vi "subUpdateTypePaletteFile.vi"(8 "error in (no error)":errorcluster, 9 "Step Types Version":string, 11 "TypePalette .ini file location":path) -> (0 "error out":errorcluster)   [LabVIEW 2015, in "veristand-steps-codegen.lvlib"]
uses:
  veristand-steps-codegen.lvlib
  <vilib>/Utility/sysdir.llb/System Directory Type.ctl
  <vilib>/xml/Load XML File.vi
  <vilib>/xml/Close Reference(Node).vi
  <vilib>/xml/Close Reference(NNMap).vi
  <vilib>/xml/NI_XML.lvlib
  <resource>/objmgr/DOMUserDefRef.rc
  <vilib>/ni/Simple XML/Simple XML.lvlib
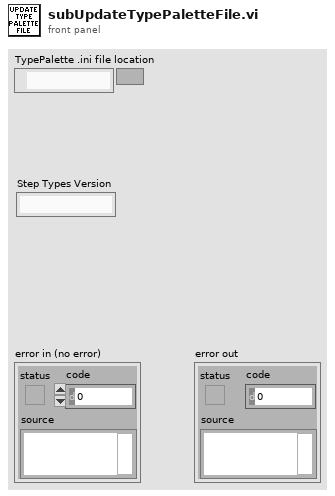
[diagram p1: front panel]
types:
  T1 = typedef "System Directory Type.ctl" = i32
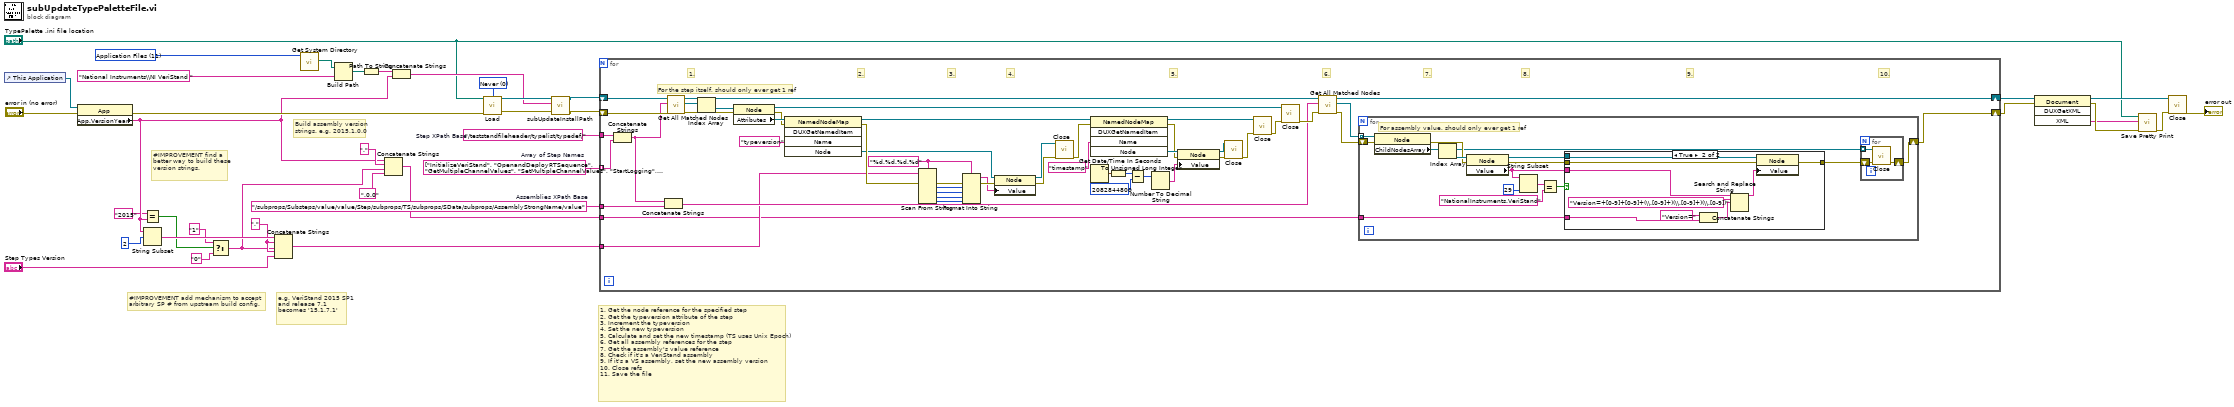
[diagram p0: block diagram]
diagram:
  w6 = "." ("string")
  w19 = T1 11 items=["User Home"=0, "User Desktop"=1, "User Documents"=2, "User Application Data"=3, "User Preferences"=4, "User Temporary"=5, "Public Documents"=6, "Public Application Data"=7, "Public Preferences"=8, "Public Cache"=13, "System Core Libraries"=9, "System Installed Libraries"=10, "Application Files"=11, "Boot Volume Root"=12] ("system directory type")
  w39 = "/subprops/Substeps/value/value/Step/subprops/TS/subprops/SData/subprops/AssemblyStrongName/value"  # Assemblies XPath Base
  w37 = string[] ["InitializeVeriStand", "OpenandDeployRTSequence", "GetMultipleChannelValues", "SetMultipleChannelValues", "StartLogging", "StopLogging", "StopVeriStand", "RunProject", "ConnectProject", "DisconnectProject", "UndeployProject", "RunStimulusProfileAsynch", "DeployProject", "OpenReferences", "GetAlarmState", "SetChannelValue", "GetAlarmList", "RunStimulusProfileBlocking", "SetAlarmState", "SetModelParameterValue", "CloseProject", "UpdateModelParametersFromFile", "GetChannelValue", "LimitTestChannelValue", "GetChannelFaultValue", "GetModelParameterValue", "ClearFault", "ClearAllFaults", "PauseRTSequence", "StopRTSequence", "GetSequenceState", "GetAllSequenceNames", "StartRTSequence", "AbortRTSequence", "GetSequenceReturnValue", "StartStimulusProfileSession", "RunRTSequenceAction", "CloseWorkspace", "OpenWorkspace", "SilentConnect", "SilentDisconnect", "OpenProject", "RunRTSequencePassFail", "RunRTSequenceNumericLimit", "SetChannelFaultValue", "StopVeristandGateway", "StartVeristand"]  # Array of Step Names
  w31 = "/teststandfileheader/typelist/typedef/"  # Step XPath Base
  w30 = 0 items=["Never", "Always", "Auto"] ("validate on load (Auto)")
  # "#IMPROVEMENT find a better way to build these version strings."
  # "Build assembly version\nstrings. e.g. 2015.1.0.0"
  # "#IMPROVEMENT add mechanism to accept\narbitrary SP # from upstream build config."
  # "e.g. VeriStand 2015 SP1 and release 7.1\nbecomes '15.1.7.1'"
  # "1. Get the node reference for the specified step\n2. Get the typeversion attribute of the step\n3. Increment the typeversion\n4. Set the new typeversion\n5. Calculate and set the new timestamp (TS uses Unix Epoch)\n6. Get all assembly references for the step\n7. Get the assembly's value reference\n8. Check if it's a VeriStand assembly\n9. If it's a VS assembly, set the new assembly version\n10. Close refs\n11. Save the file"
  n1 = control-ref of="This Application"() -> (w28:refnum<vi>)
  n2 = property class="App"(reference=w28, error in="error in (no error)") -> (error out=w14:errorcluster, "App.VersionYear"=w8:string)  [unwired: 1 out]
  n3 = String Subset(string=w8, offset (0)=2 ("length (rest)")) -> (substring=w11:string)  [unwired: 1 in]
  n4 = Equal?(x="2015", y=w8) -> (x = y?=w5:bool)
  n5 = Select(t="1" ("string"), s=w5, f="0" ("string")) -> (s? t:f=w1:string)
  n6 = Concatenate Strings(w11, w6, w1, w6, "Step Types Version") -> (w10:string)
  n7 = call <vilib>:"Get System Directory.vi"("system directory type"=w19) -> ("system directory"=w18:path)  [unwired: 10 in]
  n8 = Build Path(base path=w18, name or relative path="National Instruments\\NI VeriStand ") -> (appended path=w16:path)
  n9 = Path To String(path=w16) -> (string=w15:string)
  n10 = Concatenate Strings(w8, "." ("string"), w1, ".0.0" ("string")) -> (w24:string)
  n11 = Concatenate Strings(w15, w8) -> (w13:string)
  n12 = call-poly <vilib>:"Load.vi"("path to XML document"="TypePalette .ini file location", "validate on load (Auto)"=w30, "error in (no error)"=w14) -> ("DOM document out"=w23:refnum<k20>, "error out"=w22:errorcluster)  [unwired: 10 in, 1 out]
  n13 = call "subUpdateInstallPath.vi"("error in (no error)"=w22, "New VS InstallPath"=w13, "DOM document in"=w23) -> ("error out"=w21:errorcluster, "DOM document out"=w20:refnum<k20>)  [unwired: 7 in]
  n14 = for {
    tunnel: w37 -> [w85] mode=indexing
    shift-right: [w83] -> w32
    shift-left: w20 -> [w88]
    tunnel: w31 -> [w86]
    shift-right: [w76] -> w38
    shift-left: w21 -> [w87]
    tunnel: w39 -> [w81]
    tunnel: w10 -> [w42]
    tunnel: w24 -> [w40]
    w65 = "%d.%d.%d.%d" ("format string")
    # "10."
    # "9."
    # "8."
    # "7."
    # "6."
    # "5."
    # "4."
    # "3."
    # "2."
    # "1."
    # "For the step itself, should only ever get 1 ref"
    n15 = Concatenate Strings(w86, w85) -> (w80:string)
    n16 = Concatenate Strings(w80, w81) -> (w79:string)
    n17 = call <vilib>:"Get All Matched Nodes.vi"("error in (no error)"=w87, "XPath expression"=w80, "node in"=w88) -> ("error out"=w71:errorcluster, "node result array"=w75:refnum<k20>[], "node out"=w84:refnum<k20>)  [unwired: 6 in]
    n18 = Index Array(array=w75) -> (element=w74:refnum<k20>)  [unwired: 1 in]
    n19 = property class="Node"(reference=w74, error in=w71) -> (reference out=w49:refnum<k20>, error out=w72:errorcluster, "Attributes"=w73:refnum<k20>)
    n20 = invoke class="NamedNodeMap" method="DUXGetNamedItem"(reference=w73, error in=w72, "Name"="typeversion") -> (reference out=w64:refnum<k20>, error out=w43:errorcluster, "Node"=w41:refnum<k20>)  [unwired: 2 in, 2 out]
    n21 = Scan From String(format string=w65, input string=w42, error in=w43) -> (error out=w69:errorcluster, output 1=w68:i32, output 2=w67:i32, output 3=w66:i32, output 4=w44:i32)  [unwired: 5 in, 2 out]
    n22 = Format Into String(format string=w65, error in=w69, w68, w67, w66, w44) -> (resulting string=w62:string, error out=w63:errorcluster)  [unwired: 1 in]
    n23 = property class="Node"(reference=w41, error in=w63, "Value"=w62) -> (reference out=w60:refnum<k20>, error out=w61:errorcluster)
    n24 = call-poly <vilib>:"Close.vi"("error in (no error)"=w61, "node"=w60) -> ("error out"=w59:errorcluster)  [unwired: 7 in]
    n25 = invoke class="NamedNodeMap" method="DUXGetNamedItem"(reference=w64, error in=w59, "Name"="timestamp") -> (reference out=w52:refnum<k20>, error out=w56:errorcluster, "Node"=w57:refnum<k20>)  [unwired: 2 in, 2 out]
    n26 = Get Date/Time In Seconds() -> (seconds since 1Jan1904=w48:timestamp)
    n27 = To Unsigned Long Integer(number=w48) -> (unsigned 32bit integer=w47:u32)
    n28 = Subtract(x=w47, y=u32 2082844800) -> (x-y=w45:u32)
    n29 = Number To Decimal String(number=w45) -> (decimal integer string=w55:string)  [unwired: 1 in]
    n30 = property class="Node"(reference=w57, error in=w56, "Value"=w55) -> (reference out=w53:refnum<k20>, error out=w54:errorcluster)
    n31 = call-poly <vilib>:"Close.vi"("error in (no error)"=w54, "node"=w53) -> ("error out"=w51:errorcluster)  [unwired: 7 in]
    n32 = call-poly <vilib>:"Close.vi"("error in (no error)"=w51, "named node map"=w52) -> ("error out"=w50:errorcluster)  [unwired: 7 in]
    n33 = call-poly <vilib>:"Close.vi"("error in (no error)"=w50, "node"=w49) -> ("error out"=w82:errorcluster)  [unwired: 7 in]
    n34 = call <vilib>:"Get All Matched Nodes.vi"("error in (no error)"=w82, "XPath expression"=w79, "node in"=w84) -> ("error out"=w77:errorcluster, "node result array"=w78:refnum<k20>[], "node out"=w83:refnum<k20>)  [unwired: 6 in]
    n35 = for {
      tunnel: w78 -> [w103] mode=indexing
      shift-right: [w98] -> w76
      shift-left: w77 -> [w102]
      tunnel: w40 -> [w89]
      # "For assembly value, should only ever get 1 ref"
      n36 = property class="Node"(reference=w103, error in=w102) -> (error out=w100:errorcluster, "ChildNodesArray"=w99:refnum<k20>[])  [unwired: 1 out]
      n37 = Index Array(array=w99) -> (element=w101:refnum<k20>)  [unwired: 1 in]
      n38 = property class="Node"(reference=w101, error in=w100) -> (reference out=w95:refnum<k20>, error out=w96:errorcluster, "Value"=w94:string)
      n39 = String Subset(string=w94, length (rest)=29 ("length (rest)")) -> (substring=w92:string)  [unwired: 1 in]
      n40 = Equal?(x=w92, y="NationalInstruments.VeriStand" ("Node Value 2")) -> (x = y?=w90:bool)
      n41 = case shown="True" w90 {
        tunnel: w94 -> [_ w113]
        tunnel: [w104 w109] -> w97
        tunnel: w96 -> [w104 w107]
        tunnel: w95 -> [_ w106]
        tunnel: w89 -> [_ w105]
        frame False {
        }
        frame True {
          n42 = Concatenate Strings("Version=" ("replace string (\"\")"), w105) -> (w110:string)
          n43 = Search and Replace String(input string=w113, search string="Version=+[0-9]+[0-9]+(\\.[0-9]+)(\\.[0-9]+)(\\.[0-9])", replace string=w110) -> (result string=w108:string)  [unwired: 5 in, 3 out]
          n44 = property class="Node"(reference=w106, error in=w107, "Value"=w108) -> (error out=w109:errorcluster)  [unwired: 1 out]
        }
      }
      n45 = for {
        tunnel: w99 -> [w116] mode=indexing
        shift-right: [w114] -> w98
        shift-left: w97 -> [w115]
        n46 = call-poly <vilib>:"Close.vi"("error in (no error)"=w115, "node"=w116) -> ("error out"=w114:errorcluster)  [unwired: 7 in]
      }
    }
  }
  n47 = invoke class="Document" method="DUXGetXML"(reference=w32, error in=w38) -> (reference out=w35:refnum<k20>, error out=w34:errorcluster, "XML"=w33:string)  [unwired: 2 in, 1 out]
  n48 = call <vilib>:"Save Pretty Print.vi"("error in (no error)"=w34, "Pretty XML String"=w33, "XML file path"="TypePalette .ini file location") -> ("error out"=w36:errorcluster)  [unwired: 7 in, 1 out]
  n49 = call-poly <vilib>:"Close.vi"("error in (no error)"=w36, "node"=w35) -> ("error out"=→"error out":errorcluster)  [unwired: 7 in]
